vi "set_query infusion syringe diameter.vi"(8 "error in (no error)":errorcluster, 9 "Query?":bool, 10 "Syringe Diameter (20 mm)":dbl=4.86 min=0.0 max=99.0 format="%#.2f", 11 "VISA resource name":refnum<visa-resource-name>) -> (0 "error out":errorcluster, 2 "Output syringe diameter":string, 3 "VISA resource name out":refnum<visa-resource-name>)   [LabVIEW 2016]
doc: "Configures the syringe inside diameter (ID) in millimeters.\n\n<b>Note:</b>\n- The pump does not support remote syringe volume setting. User must set the syringe volume on the pump. \n- If you do not know the syringe diameter, refer to Appendix of the instrument manual. If your syringe is not listed on the appendix, measure the inside diameter with a vernier caliper or other precision measuring tool."
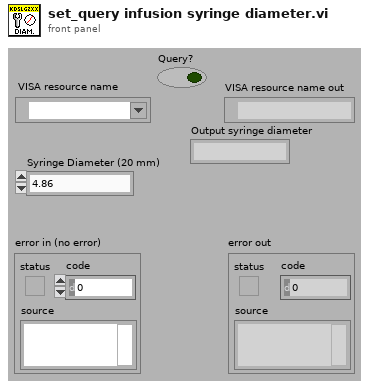
[diagram p1: front panel]
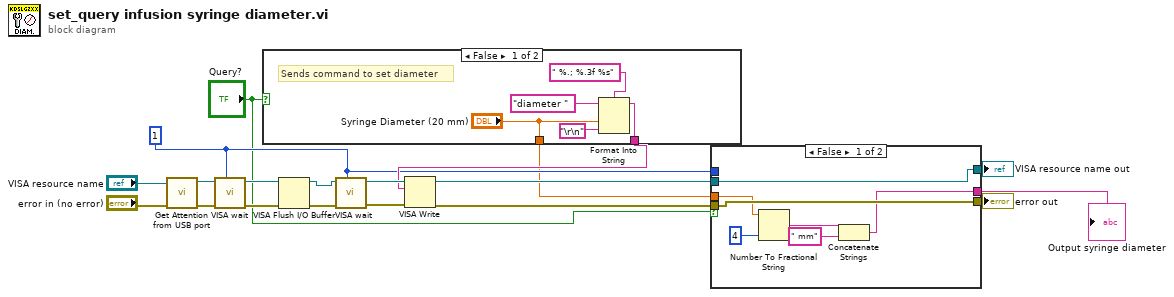
[diagram p0: block diagram]
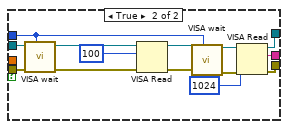
[diagram p2: hidden frame]
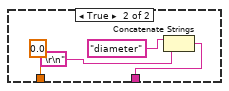
[diagram p3: hidden frame]
diagram:
  w7 = u32 1 ("milliseconds to wait")
  n1 = call "Get Attention from USB port.vi"("error in (no error)"="error in (no error)", "VISA resource name"="VISA resource name") -> ("error out"=w1:errorcluster, "VISA resource name out"=w2:refnum<visa-resource-name>)  [unwired: 8 in]
  n2 = call <userlib>:"VISA wait.vi"("VISA resource name"=w2, "error in (no error)"=w1, "milliseconds to wait"=w7) -> ("VISA resource name out"=w11:refnum<visa-resource-name>, "error out"=w10:errorcluster)  [unwired: 6 in]
  n3 = case shown="False" "Query?" {
    tunnel: [w23 w26] -> w12
    tunnel: ["Syringe Diameter (20 mm)" 0.0 ("Syringe Diameter (20 mm)")] -> w5
    frame False {
      # "Sends command to set diameter"
      n4 = Format Into String(format string=" %.; %.3f %s", initial string="diameter " ("command"), "Syringe Diameter (20 mm)", "\r\n") -> (resulting string=w23:string)  [unwired: 1 in, 1 out]
    }
    frame True {
      n5 = Concatenate Strings("diameter", "\r\n") -> (w26:string)
    }
  }
  n6 = VISA Flush I/O Buffer(VISA resource name=w11, error in (no error)=w10) -> (VISA resource name out=w9:refnum<visa-resource-name>, error out=w8:errorcluster)  [unwired: 1 in]
  n7 = call <userlib>:"VISA wait.vi"("VISA resource name"=w9, "error in (no error)"=w8, "milliseconds to wait"=w7) -> ("VISA resource name out"=w19:refnum<visa-resource-name>, "error out"=w16:errorcluster)  [unwired: 6 in]
  n8 = VISA Write(VISA resource name=w19, write buffer=w12, error in (no error)=w16) -> (VISA resource name out=w18:refnum<visa-resource-name>, error out=w17:errorcluster)  [unwired: 1 out]
  n9 = case shown="False" "Query?" {
    tunnel: w18 -> [w35 w49]
    tunnel: w17 -> [w34 w48]
    tunnel: [w35 w39] -> w15
    tunnel: [w34 w38] -> w14
    tunnel: [w30 w37] -> w13
    tunnel: w7 -> [_ w36]
    tunnel: w5 -> [w33 _]
    frame False {
      n10 = Number To Fractional String(number=w33, precision (6)=i16 4) -> (F-format string=w32:string)  [unwired: 2 in]
      n11 = Concatenate Strings(w32, " mm" ("string")) -> (w30:string)
    }
    frame True {
      n12 = call <userlib>:"VISA wait.vi"("VISA resource name"=w49, "error in (no error)"=w48, "milliseconds to wait"=w36) -> ("VISA resource name out"=w46:refnum<visa-resource-name>, "error out"=w47:errorcluster)  [unwired: 6 in]
      n13 = VISA Read(VISA resource name=w46, byte count=u32 100, error in (no error)=w47) -> (VISA resource name out=w44:refnum<visa-resource-name>, error out=w43:errorcluster)  [unwired: 2 out]
      n14 = call <userlib>:"VISA wait.vi"("VISA resource name"=w44, "error in (no error)"=w43, "milliseconds to wait"=w36) -> ("VISA resource name out"=w42:refnum<visa-resource-name>, "error out"=w41:errorcluster)  [unwired: 6 in]
      n15 = VISA Read(VISA resource name=w42, byte count=u32 1024, error in (no error)=w41) -> (VISA resource name out=w39:refnum<visa-resource-name>, read buffer=w37:string, error out=w38:errorcluster)  [unwired: 1 out]
    }
  }
  "VISA resource name out" <- w15
  "error out" <- w14
  "Output syringe diameter" <- w13
